vi "Agilent U2000 Series Configure Measurements Numbers.vi"() -> ()   [LabVIEW 2018]
doc: "This example shows how to configure the mesurements numbers for Average type in list mode.\n\nNote:\nThis VI is applicable for U2040 X-Series."
uses:
  Agilent U2000 Series.lvlib
panel:
  in  "Measurements Points (1)":i32=1
  out "Measurement":dbl
  in  "VISA resource name":refnum<visa-resource-name>
  # "(c) 2011-2015 National Instruments.  ALL RIGHTS RESERVED."
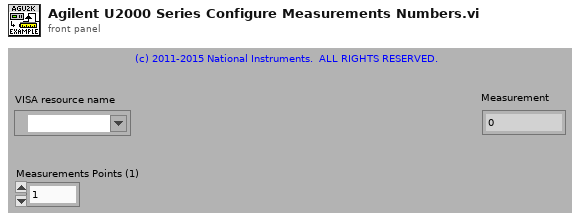
[diagram p1: front panel]
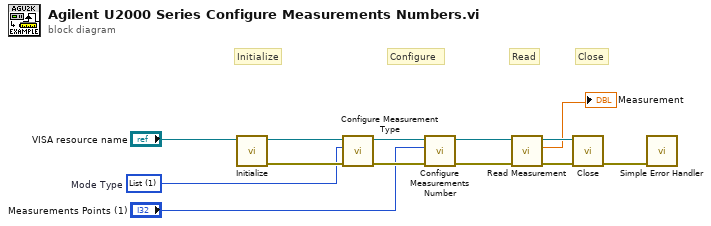
[diagram p0: block diagram]
diagram:
  w1 = 1 items=["Buffer", "List"]  # Mode Type
  # "Close"
  # "Read"
  # "Configure"
  # "Initialize"
  n1 = call "Initialize.vi"("VISA resource name"="VISA resource name") -> ("error out"=w2:errorcluster, "VISA resource name out"=w3:refnum<visa-resource-name>)  [unwired: 7 in, 2 out]
  n2 = call "Configure Measurement Type.vi"("error in (no error)"=w2, "Mode Type (0: Buffer)"=w1, "VISA resource name"=w3) -> ("error out"=w8:errorcluster, "VISA resource name out"=w9:refnum<visa-resource-name>)  [unwired: 7 in]
  n3 = call "Configure Measurements Number.vi"("error in (no error)"=w8, "Measurements Points (1)"="Measurements Points (1)", "VISA resource name"=w9) -> ("error out"=w4:errorcluster, "VISA resource name out"=w5:refnum<visa-resource-name>)  [unwired: 7 in]
  n4 = call "Read Measurement.vi"("error in (no error)"=w4, "VISA resource name"=w5) -> ("error out"=w10:errorcluster, "Measurement"=→"Measurement":dbl, "VISA resource name out"=w11:refnum<visa-resource-name>)  [unwired: 1 in, 6 out]
  n5 = call "Close.vi"("error in (no error)"=w10, "VISA resource name"=w11) -> ("error out"=w12:errorcluster)  [unwired: 9 out]
  n6 = call <vilib>:"Simple Error Handler.vi"("error in (no error)"=w12) -> ()  [unwired: 1 in, 8 out]
